vi "Wheel Separation to Frame Positions.vi"(10 "wheel separation length":dbl=1.5, 11 "wheel separation width":dbl=1.0) -> (0 "wheel y positions":dbl[](array[numeric]), 1 "wheel x positions":dbl[](array[numeric]), 2 "coerced wheel separation length":dbl, 3 "coerced wheel separation width":dbl, 4 "wheel frame angles (rad)":dbl[](array[numeric]), 6 "wheel indexes":i32[](array[numeric]))   [LabVIEW 2017, in "NI_Robotics_Mecanum Steering Frame.lvclass"]
uses:
  <vilib>/robotics/Steering/Mecanum Steering Frame/NI_Robotics_Mecanum Steering Frame.lvclass
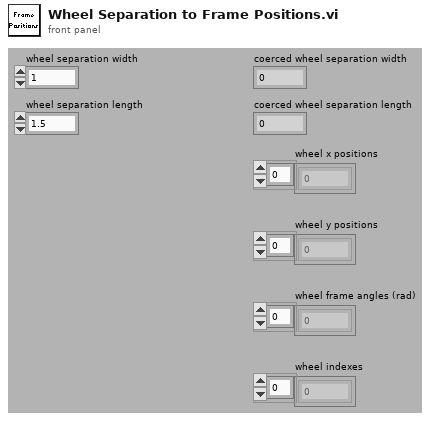
[diagram p1: front panel]
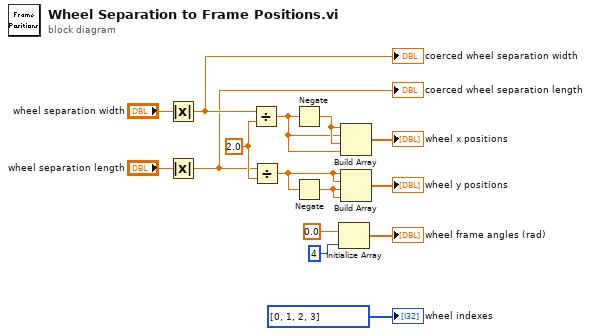
[diagram p0: block diagram]
diagram:
  w12 = 2.0 ("y")
  n1 = Absolute Value(x="wheel separation width") -> (abs(x)=w15:dbl)
  "coerced wheel separation width" <- w15
  n2 = Absolute Value(x="wheel separation length") -> (abs(x)=w1:dbl)
  "coerced wheel separation length" <- w1
  n3 = Divide(x=w15, y=w12) -> (x/y=w13:dbl)
  n4 = Divide(x=w1, y=w12) -> (x/y=w10:dbl)
  n5 = Negate(x=w13) -> (-x=w14:dbl)
  n6 = Negate(x=w10) -> (-x=w11:dbl)
  n7 = Initialize Array(0.0 ("element"), 4 ("dimension size")) -> (→"wheel frame angles (rad)":dbl[])
  n8 = Build Array(w14, w13, w14, w13) -> (→"wheel x positions":dbl[])
  n9 = Build Array(w10, w10, w11, w11) -> (→"wheel y positions":dbl[])
  "wheel indexes" <- i32[] [0, 1, 2, 3] ("wheel indexes")
